vi "init.vi"(0 "UART port in":T1) -> (1 "error out":errorcluster, 2 "UART port out":T1)   [LabVIEW 2010]
uses:
  UART/UART Port Type.ctl
  Open Interface Controls/iRobot Sensor ID.ctl
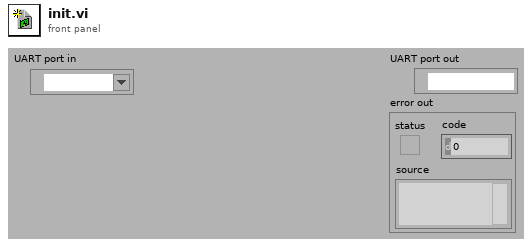
[diagram p1: front panel]
types:
  T1 = typedef "UART Port Type.ctl" = refnum<visa-resource-name>
  T2 = typedef "iRobot Sensor ID.ctl" = enum8{"Sensor Group 0", "Sensor Group 1", "Sensor Group 2", "Sensor Group 3", "Sensor Group 4", "Sensor Group 5", "Sensor Group 6", "Bump + Wheel Drop", "Wall", "Cliff Left", "Cliff Front Left", "Cliff Front Right", "Cliff Right", "Virtual Wall", "Low Side Driver + Wheel Overcurrent", "Unused 0", "Unused 1", "Infrared", "Buttons", "Distance", "Angle", "Charging State", "Voltage", "Current", "Battery Temperature", "Battery Charge", "Battery Capacity", "Wall Signal", "Cliff Left Signal", "Cliff Front Left Signal", "Cliff Front Right Signal", "Cliff Right Signal", "Cargo Bay Digital Inputs", "Cargo Bay Analog Signal", "Charging Sources Available", "OI Mode", "Song Number", "Song Playing", "Number of Stream Packets", "Requested Velocity", "Requested Radius", "Requested Right Velocity", "Requested Left Velocity"}
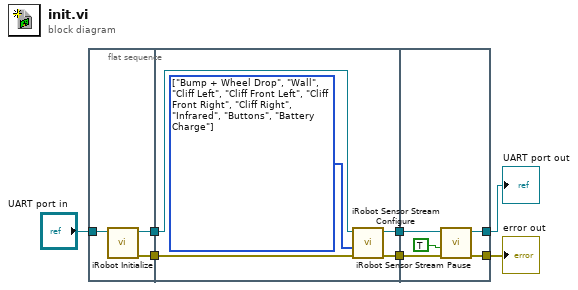
[diagram p0: block diagram]
diagram:
  n1 = flat-sequence {
    tunnel: "UART port in" -> [w10]
    tunnel: [w9] -> w6
    tunnel: [w8] -> w4
    tunnel: w6 -> [w15]
    tunnel: [w14] -> w5
    tunnel: w4 -> [w12]
    tunnel: [w11] -> w3
    tunnel: w5 -> [w20]
    tunnel: w3 -> [w18]
    tunnel: [w17] -> w2
    tunnel: [w16] -> w1
    frame #0 {
      n2 = call "iRobot Initialize.vi"("UART port in"=w10) -> ("error out"=w8:errorcluster, "UART port out"=w9:T1)  [unwired: 9 in]
    }
    frame #1 {
      w13 = T2[] [enum."Bump + Wheel Drop", enum."Wall", enum."Cliff Left", enum."Cliff Front Left", enum."Cliff Front Right", enum."Cliff Right", enum."Infrared", enum."Buttons", enum."Battery Charge"] items=["Sensor Group 0", "Sensor Group 1", "Sensor Group 2", "Sensor Group 3", "Sensor Group 4", "Sensor Group 5", "Sensor Group 6", "Bump + Wheel Drop", "Wall", "Cliff Left", "Cliff Front Left", "Cliff Front Right", "Cliff Right", "Virtual Wall", "Low Side Driver + Wheel Overcurrent", "Unused 0", "Unused 1", "Infrared", "Buttons", "Distance", "Angle", "Charging State", "Voltage", "Current", "Battery Temperature", "Battery Charge", "Battery Capacity", "Wall Signal", "Cliff Left Signal", "Cliff Front Left Signal", "Cliff Front Right Signal", "Cliff Right Signal", "Cargo Bay Digital Inputs", "Cargo Bay Analog Signal", "Charging Sources Available", "OI Mode", "Song Number", "Song Playing", "Number of Stream Packets", "Requested Velocity", "Requested Radius", "Requested Right Velocity", "Requested Left Velocity"] ("Sensors")
      n3 = call "iRobot Sensor Stream Configure.vi"("error in"=w12, "Sensors"=w13, "UART port in"=w15) -> ("error out"=w11:errorcluster, "UART port out"=w14:T1)  [unwired: 7 in]
    }
    frame #2 {
      n4 = call "iRobot Sensor Stream Pause.vi"("error in"=w18, "Resume?"=TRUE, "UART port in"=w20) -> ("error out"=w16:errorcluster, "UART port out"=w17:T1)  [unwired: 7 in]
    }
  }
  "UART port out" <- w2
  "error out" <- w1
